vi "ni579x Store Characterization Data (EEPROM).vi"(0 "Register Bus":refnum<class "ni579x Register Bus v1 Host.lvclass">=refnum, 1 "scope":string(combo)="characterization data eeprom", 2 "EEPROM Header":T7={"Checksum"=0, "Product Code"=30298, "Hardware Current Version"=1, "Hardware Oldest Compatible Version"=1, "EEPROM Map Current Version"=0, "EEPROM Map Oldest Compatible Version"=0, "User Password"="", "Pointer to Factory Header"=64, "Pointer to User Header"=0, "Recommended Interval"=12, "Number of Reserved Bytes"=32} {"Product Code" format="%x"; "Checksum" format="%x"}, 5 "EEPROM Calibration Header":T6={"Checksum"=0, "Date"=timestamp(0 s since 1904-01-01), "Temperature"=25.0, "Misc. Info"="", "Pointer to Device Data Header"=128, "Number of Reserved Bytes"=28} {"Checksum" format="%x"}, 7 "Device Data Header":T5={"Checksum"=0, "Number of Channels"=2, "Number of Attenuations"=[255, 128], "Number of Attenuator Settings"=[2, 1], "Number of Gain Settings"=[64, 32], "Pointer to Cal Data"=[160, 68546], "Number of Reserved Bytes"=7, "Number of Frequencies"=[168, 168]} {"Checksum" format="%x"}, 9 "Characterization Data":T2[](array[typedef]) {"Frequencies [Hz]" format="%#_6p"}, 11 "Error In":errorcluster, 12 "start address":u32 format="%x", 13 "EEPROM Data Section":T1) -> (4 "Register Bus (out)":refnum<class "ni579x Register Bus v1 Host.lvclass">, 15 "Error Out":errorcluster)   [LabVIEW 2013]
doc: "Stores headers and per-channel characterization data in the on-device EEPROM.\nWARNING: THIS WILL ERASE EXISTING DATA IN THE EEPROM. CONTACT NATIONAL INSTRUMENTS BEFORE USING THIS VI.\n\n<B>Input Parameters</B>\n\n<B>Register Bus</B> The Register Bus object created by the ni579x Open VI and used as the session handle for the NI-579x Configuration Design Library.\n\n<B>scope</B> The EEPROM to read characterization data from. The only option is \"characterization data eeprom\".\n\n<B>start address</B> The start offset of the data in the EEPROM.\n\n<B>EEPROM Data Section</B> The EEPROM can contain characterization data measured and calculated by the manufacturer (the Factory Data) as well as data measured and calculated by the user (the User Data).\nNOTE: YOU SHOULD NEVER WRITE TO THE FACTORY DATA.\n\n<B>EEPROM Header</B> Header information for the entire EEPROM.\n\n<B>EEPROM Calibration Header</B> Header information describing the calibration sections.\n\n<B>Device Data Header</B> Header information describing the device characterization data sections.\n\n<B>Characterization Data</B> An array of characterization data for each channel.\nFor the 5791,\n the Rx channel is index 0\n the Tx channel is index 1\n\n<B>Output Parameters</B>\n\n<B>Register Bus (out)</B> The Register Bus object created by the ni579x Open VI and used as the session handle for the NI-579x Configuration Design Library."
uses:
  <instrlib>/ni579x/Register Bus/v1/Host/ni579x Register Bus v1 Host.lvclass
  <instrlib>/ni579x/Config/v1/Shared/Types/EEPROM/ni579x EEPROM Header.ctl
  <instrlib>/ni579x/Config/v1/Shared/Types/EEPROM/ni579x EEPROM Calibration Header.ctl
  <instrlib>/ni579x/Config/v1/Shared/Types/EEPROM/ni579x EEPROM Device Data Header.ctl
  <instrlib>/ni579x/Config/v1/Shared/Types/ni579x Characterization Data.ctl
  <instrlib>/ni579x/Config/v1/Shared/Types/ni579x IQ Imbalance.ctl
  <instrlib>/ni579x/Config/v1/Shared/Types/ni579x Gain to Attenuation Mapping.ctl
  <instrlib>/ni579x/Config/v1/Shared/Types/EEPROM/ni579x EEPROM Data Section.ctl
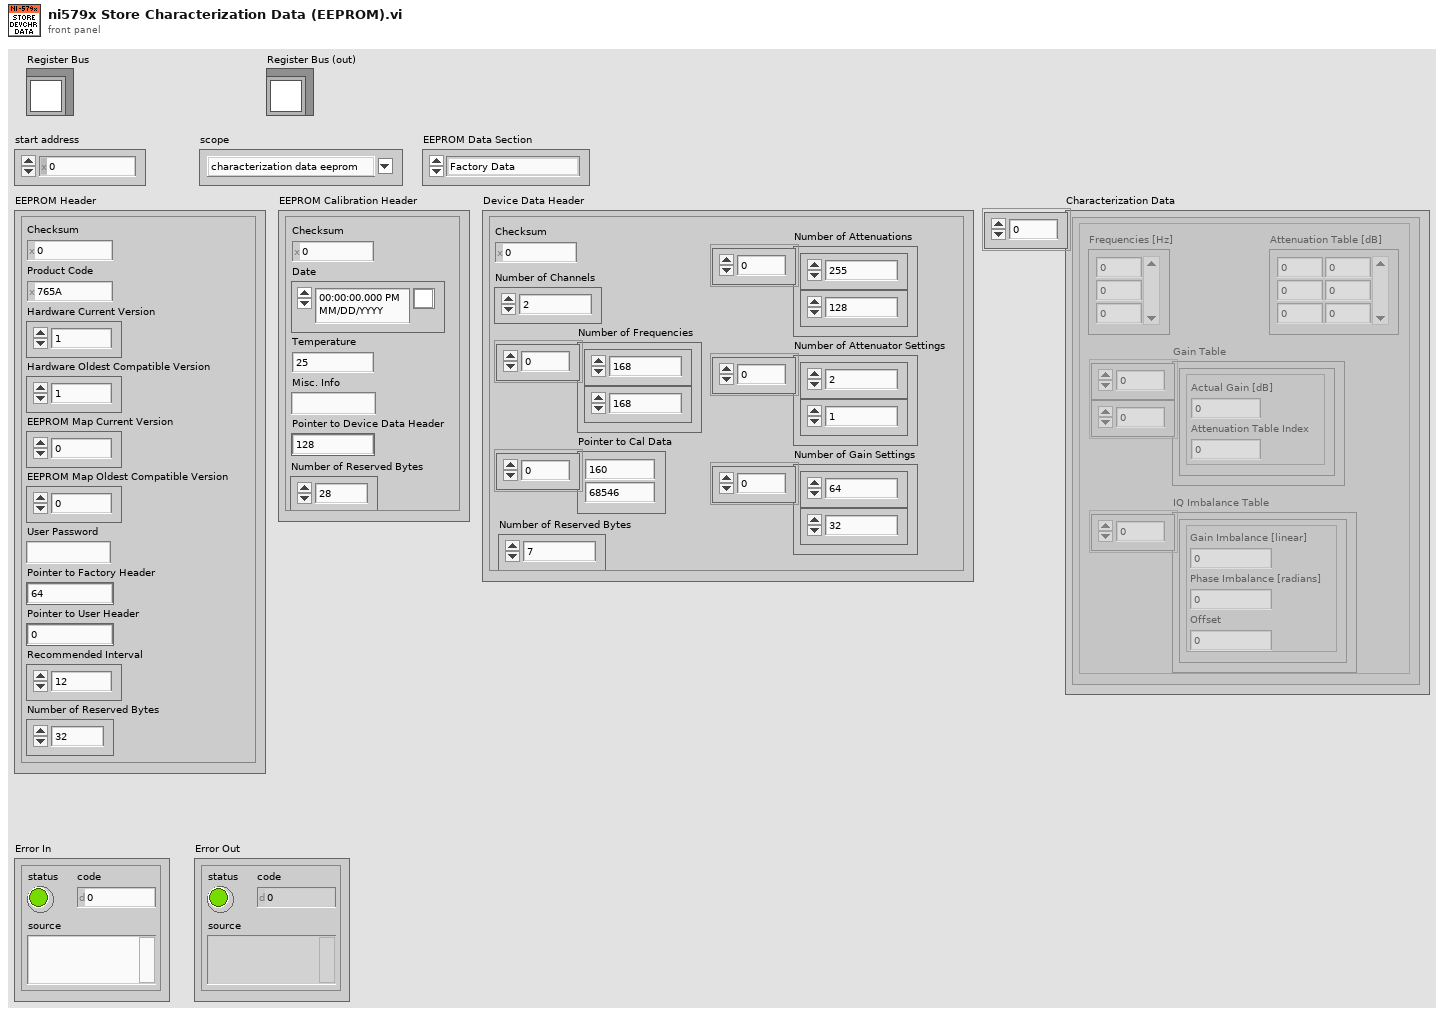
[diagram p1: front panel]
types:
  T1 = typedef "ni579x EEPROM Data Section.ctl" = enum16{"Factory Data", "User Data"}
  T2 = typedef "ni579x Characterization Data.ctl" = cluster{"Attenuation Table [dB]":dbl[][], "Frequencies [Hz]":dbl[], "IQ Imbalance Table":T3[], "Gain Table":T4[][]}
  T3 = typedef "ni579x IQ Imbalance.ctl" = cluster{"Gain Imbalance [linear]":dbl, "Phase Imbalance [radians]":dbl, "Offset":cdb}
  T4 = typedef "ni579x Gain to Attenuation Mapping.ctl" = cluster{"Actual Gain [dB]":dbl, "Attenuation Table Index":i32}
  T5 = typedef "ni579x EEPROM Device Data Header.ctl" = cluster{"Checksum":u32, "Number of Channels":u8, "Number of Attenuations":u16[], "Number of Attenuator Settings":u8[], "Number of Gain Settings":u8[], "Pointer to Cal Data":u32[], "Number of Reserved Bytes":i32, "Number of Frequencies":u16[]}
  T6 = typedef "ni579x EEPROM Calibration Header.ctl" = cluster{"Checksum":u32, "Date":timestamp, "Temperature":sgl, "Misc. Info":string, "Pointer to Device Data Header":u32, "Number of Reserved Bytes":i32}
  T7 = typedef "ni579x EEPROM Header.ctl" = cluster{"Checksum":u32, "Product Code":u16, "Hardware Current Version":u16, "Hardware Oldest Compatible Version":u16, "EEPROM Map Current Version":u16, "EEPROM Map Oldest Compatible Version":u16, "User Password":string, "Pointer to Factory Header":u32, "Pointer to User Header":u32, "Recommended Interval":u16, "Number of Reserved Bytes":i32}
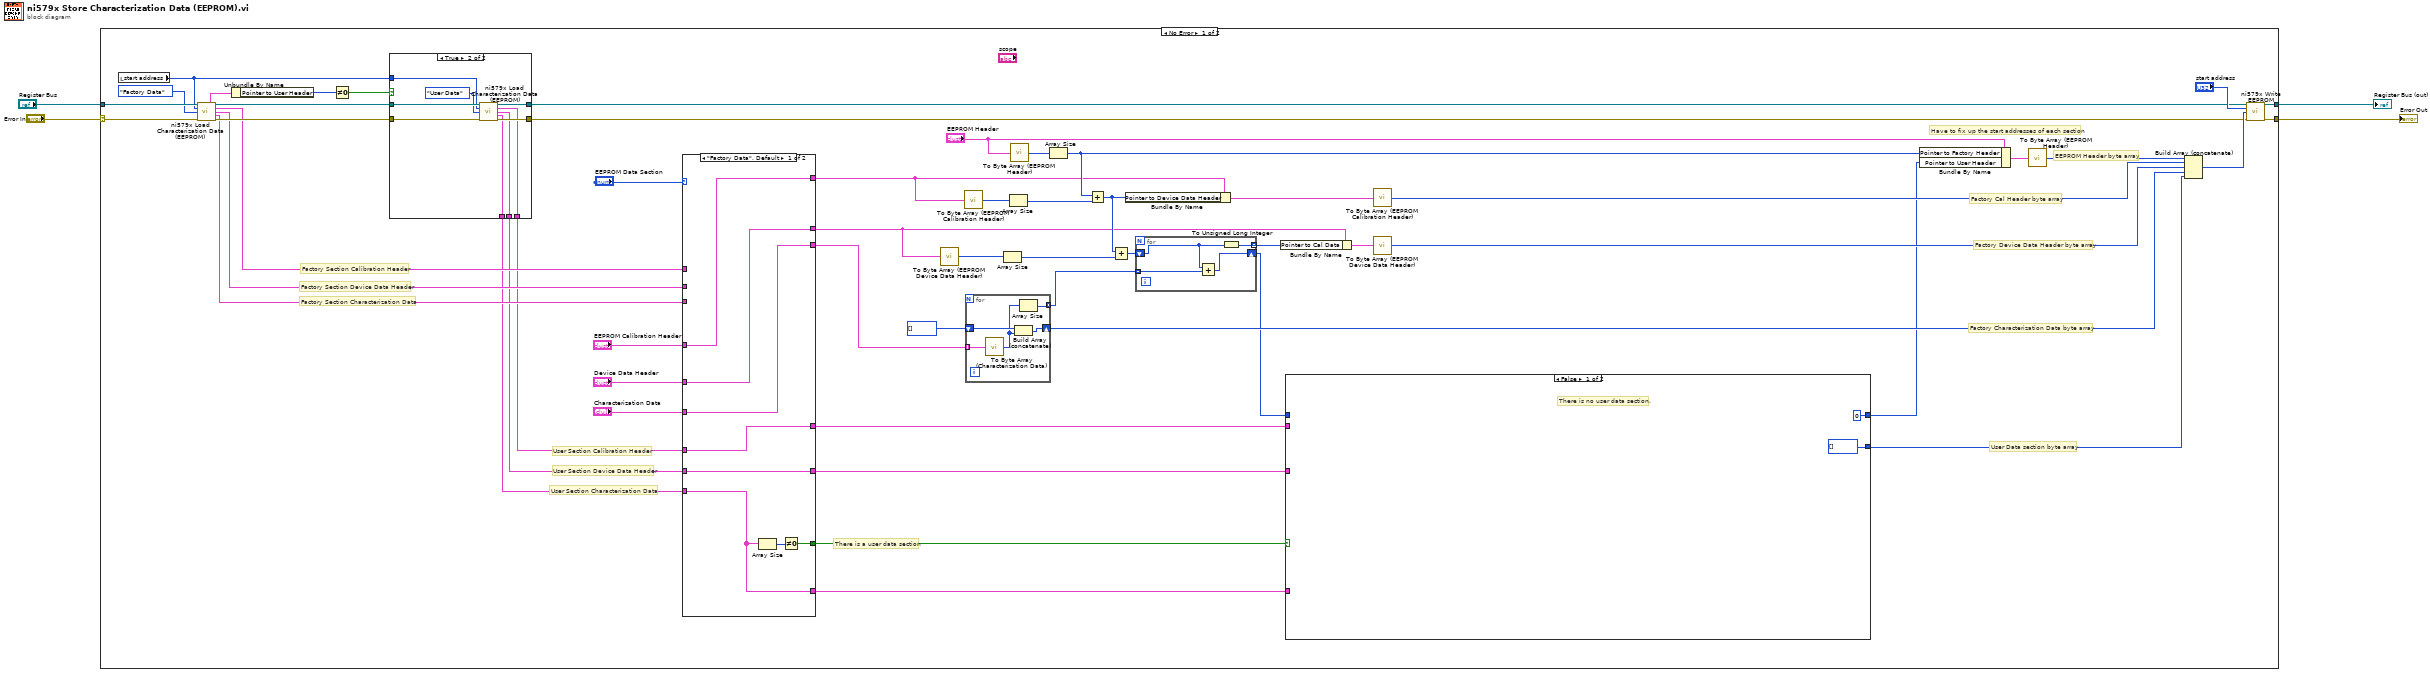
[diagram p0: block diagram]
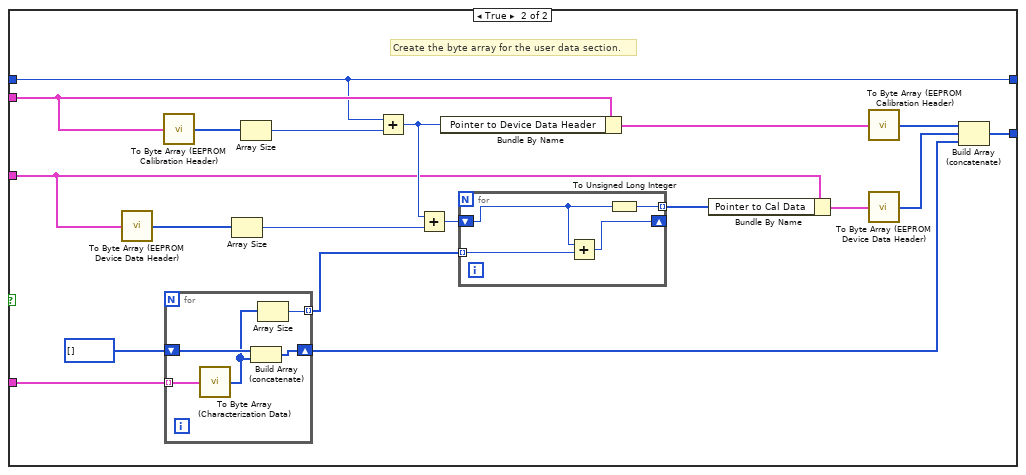
[diagram p2: hidden frame]
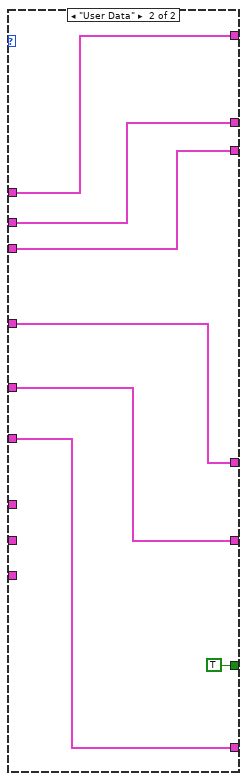
[diagram p3: hidden frame]
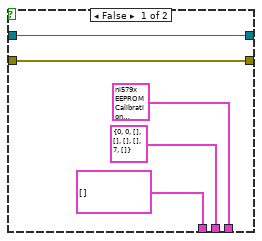
[diagram p4: hidden frame]
diagram:
  n1 = case shown="No Error" "Error In" {
    selector: "Error In" -> [w34 w128]
    tunnel: [w57 w128] -> w3
    tunnel: "Register Bus" -> [w35 w127]
    tunnel: [w58 w127] -> w1
    frame No Error {
      # "Factory Cal Header byte array"
      # "Factory Characterization Data byte array"
      # "Factory Device Data Header byte array"
      # "EEPROM Header byte array"
      # "User Data section byte array"
      # "There is a user data section"
      # "User Section Characterization Data"
      # "User Section Device Data Header"
      # "User Section Calibration Header"
      # "Factory Section Characterization Data"
      # "Factory Section Device Data Header"
      # "Factory Section Calibration Header"
      # "Have to fix up the start addresses of each section"
      n2 = local read "start address"() -> (w30:u32)
      n3 = call <instrlib>:"ni579x Load Characterization Data (EEPROM).vi"("Register Bus"=w35, "start address"=w30, "EEPROM Data Section"=ni579x_EEPROM_Data_Section."Factory Data", "Error In"=w34) -> ("EEPROM Header"=w29:T7, "Register Bus (out)"=w31:refnum<class "ni579x Register Bus v1 Host.lvclass">, "EEPROM Calibration Header"=w19:T6, "Device Data Header"=w18:T5, "Characterization Data"=w17:T2[], "Error Out"=w33:errorcluster)  [unwired: 6 in]
      n4 = Unbundle By Name(w29) -> ("Pointer to User Header"=w28:u32)
      n5 = Not Equal To 0?(x=w28) -> (x != 0?=w27:bool)
      n6 = case shown="True" w27 {
        tunnel: w33 -> [w104 w117]
        tunnel: w31 -> [w105 w116]
        tunnel: w30 -> [_ w115]
        tunnel: [w105 w113] -> w6
        tunnel: [w104 w112] -> w5
        tunnel: [T6 {"Checksum"=0, "Date"=timestamp(0 s since 1904-01-01), "Temperature"=0.0, "Misc. Info"="", "Pointer to Device Data Header"=0, "Number of Reserved Bytes"=28} ("EEPROM Calibration Header") w111] -> w13
        tunnel: [T5 {"Checksum"=0, "Number of Channels"=0, "Number of Attenuations"=[], "Number of Attenuator Settings"=[], "Number of Gain Settings"=[], "Pointer to Cal Data"=[], "Number of Reserved Bytes"=7, "Number of Frequencies"=[]} ("Device Data Header") w110] -> w12
        tunnel: [T2[] [] ("Characterization Data") w109] -> w11
        frame False {
        }
        frame True {
          n7 = call <instrlib>:"ni579x Load Characterization Data (EEPROM).vi"("Register Bus"=w116, "start address"=w115, "EEPROM Data Section"=ni579x_EEPROM_Data_Section."User Data", "Error In"=w117) -> ("Register Bus (out)"=w113:refnum<class "ni579x Register Bus v1 Host.lvclass">, "EEPROM Calibration Header"=w111:T6, "Device Data Header"=w110:T5, "Characterization Data"=w109:T2[], "Error Out"=w112:errorcluster)  [unwired: 6 in, 1 out]
        }
      }
      n8 = case shown="\"Factory Data\", Default" "EEPROM Data Section" {
        tunnel: [w96 w103] -> w25
        tunnel: "EEPROM Calibration Header" -> [w96 w100]
        tunnel: [w95 w102] -> w23
        tunnel: "Device Data Header" -> [w95 w98]
        tunnel: [w94 w101] -> w21
        tunnel: "Characterization Data" -> [w94 w99]
        tunnel: w19 -> [_ w103]
        tunnel: w18 -> [_ w102]
        tunnel: w17 -> [_ w101]
        tunnel: [w93 w100] -> w16
        tunnel: [w91 w99] -> w15
        tunnel: [w92 w98] -> w14
        tunnel: w13 -> [w93 _]
        tunnel: w12 -> [w92 _]
        tunnel: w11 -> [w91 _]
        tunnel: [w89 TRUE] -> w10
        frame "Factory Data", Default {
          n9 = Array Size(array=w91) -> (size(s)=w90:i32)
          n10 = Not Equal To 0?(x=w90) -> (x != 0?=w89:bool)
        }
        frame "User Data" {
        }
      }
      n11 = call <instrlib>:"To Byte Array (EEPROM Device Data Header).vi"("Device Data Header"=w23) -> ("byte array out"=w47:u8[])
      n12 = call <instrlib>:"To Byte Array (EEPROM Calibration Header).vi"("EEPROM Calibration Header"=w25) -> ("byte array out"=w51:u8[])
      n13 = for {
        tunnel: w21 -> [w126] mode=indexing
        shift-right: [w125] -> w54
        shift-left: u8[] [] -> [w124]
        tunnel: [w122] -> w46 mode=indexing
        n14 = call <instrlib>:"To Byte Array (Characterization Data).vi"("Characterization Data"=w126) -> ("byte array out"=w123:u8[])
        n15 = Build Array (concatenate)(w124, w123) -> (w125:u8[])
        n16 = Array Size(array=w123) -> (size(s)=w122:i32)
      }
      n17 = Array Size(array=w47) -> (size(s)=w45:i32)
      n18 = Array Size(array=w51) -> (size(s)=w48:i32)
      n19 = call <instrlib>:"To Byte Array (EEPROM Header).vi"("EEPROM Header"="EEPROM Header") -> ("byte array out"=w52:u8[])
      n20 = Array Size(array=w52) -> (size(s)=w49:i32)
      n21 = Add(x=w49, y=w48) -> (x+y=w44:i32)
      n22 = Add(x=w44, y=w45) -> (x+y=w43:i32)
      n23 = Bundle By Name(cluster=w25, "Pointer to Device Data Header"=w44) -> (w39:T6)
      n24 = for {
        tunnel: w46 -> [w121] mode=indexing
        shift-right: [w119] -> w9
        shift-left: w43 -> [w120]
        tunnel: [w118] -> w42 mode=indexing
        n25 = Add(x=w120, y=w121) -> (x+y=w119:i32)
        n26 = To Unsigned Long Integer(number=w120) -> (unsigned 32bit integer=w118:u32)
      }
      n27 = Bundle By Name(cluster=w23, "Pointer to Cal Data"=w42) -> (w38:T5)
      n28 = case shown="False" w10 {
        tunnel: w16 -> [_ w66]
        tunnel: w15 -> [_ w68]
        tunnel: w14 -> [_ w67]
        tunnel: w9 -> [_ w61]
        tunnel: [u8[] [] w62] -> w8
        tunnel: [0 w61] -> w7
        frame False {
          # "There is no user data section."
        }
        frame True {
          # "Create the byte array for the user data section."
          n29 = call <instrlib>:"To Byte Array (EEPROM Device Data Header).vi"("Device Data Header"=w67) -> ("byte array out"=w72:u8[])
          n30 = call <instrlib>:"To Byte Array (EEPROM Calibration Header).vi"("EEPROM Calibration Header"=w66) -> ("byte array out"=w70:u8[])
          n31 = for {
            tunnel: w68 -> [w88] mode=indexing
            shift-right: [w87] -> w63
            shift-left: u8[] [] -> [w86]
            tunnel: [w84] -> w73 mode=indexing
            n32 = call <instrlib>:"To Byte Array (Characterization Data).vi"("Characterization Data"=w88) -> ("byte array out"=w85:u8[])
            n33 = Build Array (concatenate)(w86, w85) -> (w87:u8[])
            n34 = Array Size(array=w85) -> (size(s)=w84:i32)
          }
          n35 = Array Size(array=w72) -> (size(s)=w74:i32)
          n36 = Array Size(array=w70) -> (size(s)=w71:i32)
          n37 = Add(x=w61, y=w71) -> (x+y=w75:i32)
          n38 = Add(x=w75, y=w74) -> (x+y=w76:i32)
          n39 = Bundle By Name(cluster=w66, "Pointer to Device Data Header"=w75) -> (w78:T6)
          n40 = for {
            tunnel: w73 -> [w83] mode=indexing
            shift-right: [w81] -> _
            shift-left: w76 -> [w82]
            tunnel: [w80] -> w77 mode=indexing
            n41 = Add(x=w82, y=w83) -> (x+y=w81:i32)
            n42 = To Unsigned Long Integer(number=w82) -> (unsigned 32bit integer=w80:u32)
          }
          n43 = Bundle By Name(cluster=w67, "Pointer to Cal Data"=w77) -> (w79:T5)
          n44 = call <instrlib>:"To Byte Array (EEPROM Calibration Header).vi"("EEPROM Calibration Header"=w78) -> ("byte array out"=w65:u8[])
          n45 = call <instrlib>:"To Byte Array (EEPROM Device Data Header).vi"("Device Data Header"=w79) -> ("byte array out"=w64:u8[])
          n46 = Build Array (concatenate)(w65, w64, w63) -> (w62:u8[])
        }
      }
      n47 = call <instrlib>:"To Byte Array (EEPROM Calibration Header).vi"("EEPROM Calibration Header"=w39) -> ("byte array out"=w37:u8[])
      n48 = call <instrlib>:"To Byte Array (EEPROM Device Data Header).vi"("Device Data Header"=w38) -> ("byte array out"=w36:u8[])
      n49 = Bundle By Name(cluster="EEPROM Header", "Pointer to Factory Header"=w49, "Pointer to User Header"=w7) -> (w41:T7)
      n50 = call <instrlib>:"To Byte Array (EEPROM Header).vi"("EEPROM Header"=w41) -> ("byte array out"=w40:u8[])
      n51 = Build Array (concatenate)(w40, w37, w36, w54, w8) -> (w53:u8[])
      n52 = call <instrlib>:"ni579x Write EEPROM.vi"("Register Bus"=w6, "start address"="start address", "data"=w53, "Error In"=w5) -> ("Register Bus (out)"=w58:refnum<class "ni579x Register Bus v1 Host.lvclass">, "Error Out"=w57:errorcluster)  [unwired: 10 in]
    }
    frame Error {
    }
  }
  "Register Bus (out)" <- w1
  "Error Out" <- w3
